vi "未命名 3.vi"(1 "b":dbl, 2 "k":dbl, 3 "x":dbl) -> (0 "y":dbl)   [LabVIEW 2017]
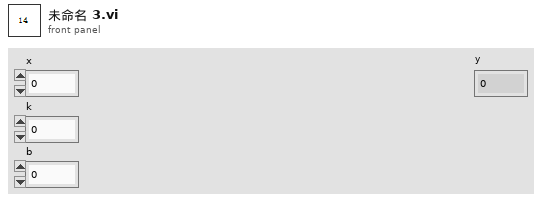
[diagram p1: front panel]
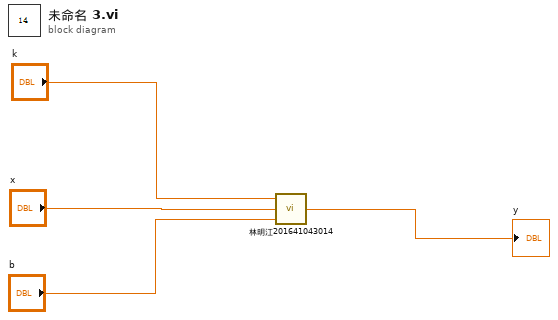
[diagram p0: block diagram]
diagram:
  n1 = call "林明江201641043014.vi"("b"="b", "x"="x", "k"="k") -> ("4"=→"y":dbl)
